vi "1D Fit Effective Number of Parameters.vi"(2 "parameter bounds":T1) -> (7 "Effective Number of Parameters":i32)   [LabVIEW 2021, in "Fits.lvlib"]
uses:
  Fits.lvlib
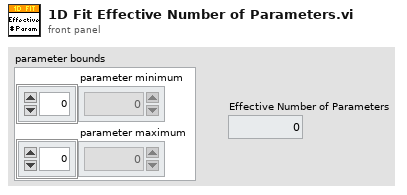
[diagram p1: front panel]
types:
  T1 = cluster{"parameter minimum":dbl[], "parameter maximum":dbl[]}
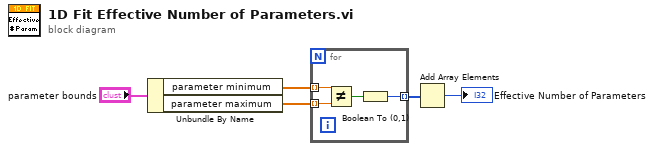
[diagram p0: block diagram]
diagram:
  n1 = Unbundle By Name("parameter bounds") -> ("parameter minimum"=w4:dbl[], "parameter maximum"=w3:dbl[])
  n2 = for {
    tunnel: w4 -> [w9] mode=indexing
    tunnel: w3 -> [w8] mode=indexing
    tunnel: [w6] -> w2 mode=indexing
    n3 = Not Equal?(x=w9, y=w8) -> (x != y?=w7:bool)
    n4 = Boolean To (0,1)(Boolean=w7) -> (0, 1=w6:i16)
  }
  n5 = Add Array Elements(numeric array=w2) -> (sum=→"Effective Number of Parameters":i16)
